vi "Test Flatten to Path.vi"() -> ()   [LabVIEW 2017]
uses:
  c9b6f366-5878-41eb-ba35-ba660d6be02e.vi
  Variant to JSON Text.vi
  JSONtext.lvlib
  <vilib>/addons/_JKI Toolkits/Caraya/classes/Test/Test.lvclass
  <vilib>/addons/_JKI Toolkits/Caraya/classes/Assert/Assert.lvclass
panel:
  out "$Paths":string[](array[string])
  out "<JSON>":string
  out "JSON recovered":bool
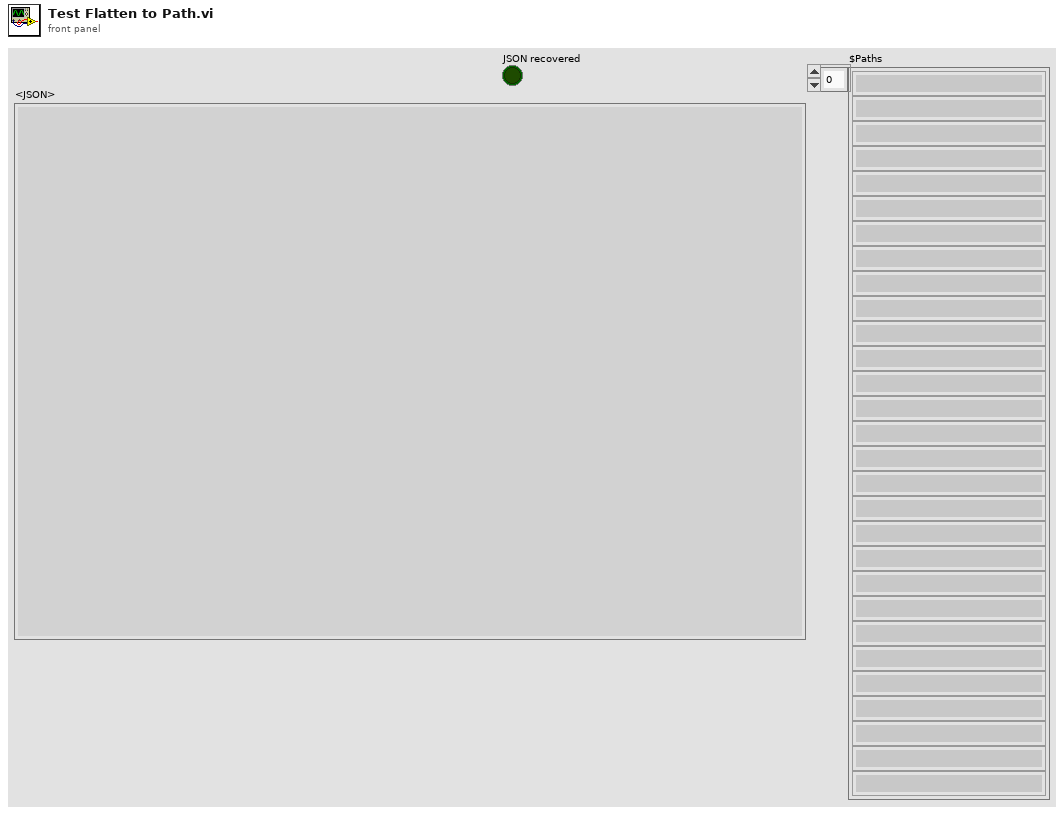
[diagram p1: front panel]
types:
  T1 = cluster{"Number":i32, "String":string, "Timestamp":timestamp, "Reply refnum":refnum<queue>, "VISA resource name":refnum<visa-resource-name>, "True":bool, "Enum":enum16{"Enum 1", "Enum 22", "Enum 333"}, "DBL":dbl, "SubC":cluster{"Number":i32, "String":string, "Timestamp":timestamp, "Reply refnum":refnum<queue>, "VISA resource name":refnum<visa-resource-name>, "True":bool, "Enum":enum16{"Enum 1", "Enum 22", "Enum 333"}, "DBL":dbl, "SubC":cluster{"Number":i32, "String":string, "Timestamp":timestamp, "Reply refnum":refnum<queue>, "VISA resource name":refnum<visa-resource-name>, "True":bool, "Enum":enum16{"Enum 1", "Enum 22", "Enum 333"}, "DBL":dbl}}}
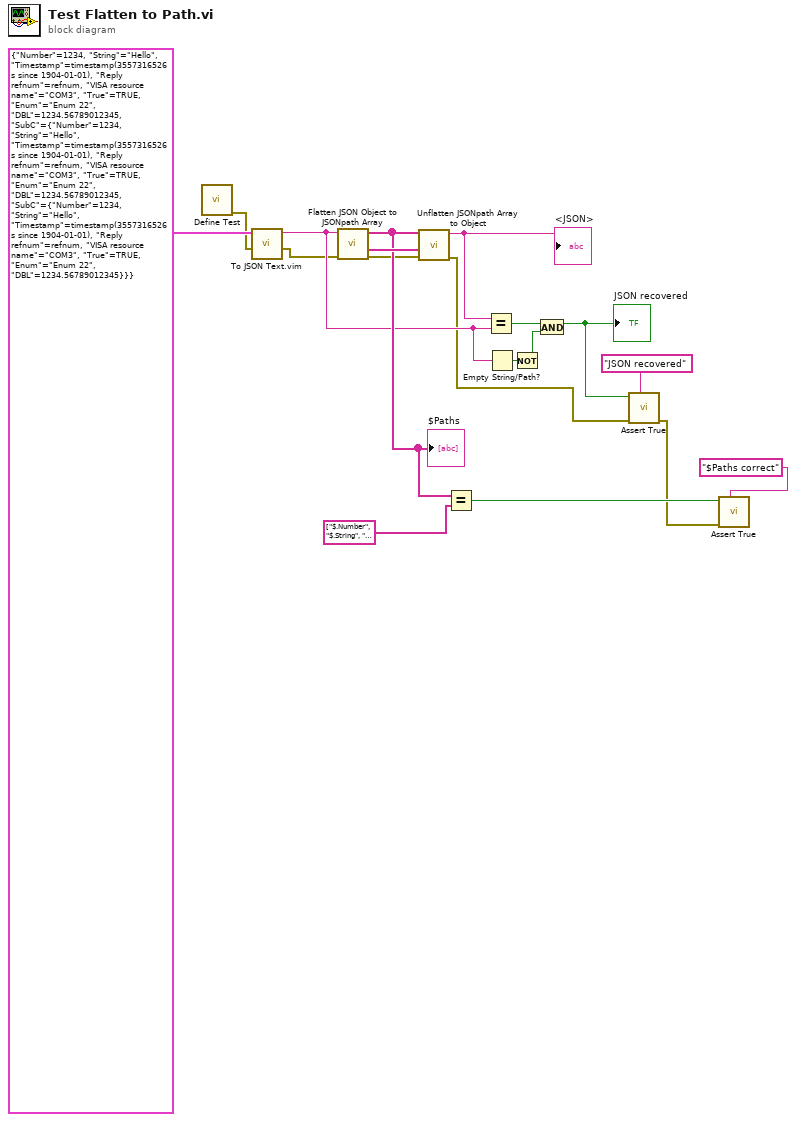
[diagram p0: block diagram]
diagram:
  n1 = call <vilib>:"Define Test.vi"() -> ("error out"=w2:errorcluster)  [unwired: 11 in]
  n2 = call "To JSON Text.vim"("error in (no error)"=w2, "Anything"=T1 {"Number"=1234, "String"="Hello", "Timestamp"=timestamp(3557316526.864 s since 1904-01-01), "Reply refnum"=refnum, "VISA resource name"="COM3", "True"=TRUE, "Enum"=enum."Enum 22", "DBL"=1234.56789012345, "SubC"={"Number"=1234, "String"="Hello", "Timestamp"=timestamp(3557316526.864 s since 1904-01-01), "Reply refnum"=refnum, "VISA resource name"="COM3", "True"=TRUE, "Enum"=enum."Enum 22", "DBL"=1234.56789012345, "SubC"={"Number"=1234, "String"="Hello", "Timestamp"=timestamp(3557316526.864 s since 1904-01-01), "Reply refnum"=refnum, "VISA resource name"="COM3", "True"=TRUE, "Enum"=enum."Enum 22", "DBL"=1234.56789012345}}}) -> ("error out"=w5:errorcluster, "<JSON>"=w12:string)  [unwired: 8 in]
  n3 = call "Flatten JSON Object to JSONpath Array.vi"("error in (no error)"=w5, "JSON"=w12) -> ("error out"=w4:errorcluster, "<JSON>"=w15:string[], "$Paths"=w14:string[])  [unwired: 7 in]
  "$Paths" <- w14
  n4 = call "Unflatten JSONpath Array to Object.vi"("error in (no error)"=w4, "JSON Items"=w15, "$Paths"=w14) -> ("error out"=w3:errorcluster, "<JSON>"=w17:string)  [unwired: 7 in]
  "<JSON>" <- w17
  n5 = Equal?(x=w14, y=string[] ["$.Number", "$.String", "$.Timestamp", "$.Reply refnum", "$.VISA resource name", "$.True", "$.Enum", "$.DBL", "$.SubC.Number", "$.SubC.String", "$.SubC.Timestamp", "$.SubC.Reply refnum", "$.SubC.VISA resource name", "$.SubC.True", "$.SubC.Enum", "$.SubC.DBL", "$.SubC.SubC.Number", "$.SubC.SubC.String", "$.SubC.SubC.Timestamp", "$.SubC.SubC.Reply refnum", "$.SubC.SubC.VISA resource name", "$.SubC.SubC.True", "$.SubC.SubC.Enum", "$.SubC.SubC.DBL"] ("$Paths")) -> (x = y?=w7:bool)
  n6 = Equal?(x=w17, y=w12) -> (x = y?=w16:bool)
  n7 = Empty String/Path?(string/path=w12) -> (empty?=w10:bool)
  n8 = Not(x=w10) -> (.not. x?=w11:bool)
  n9 = And(x=w16, y=w11) -> (x .and. y?=w8:bool)
  "JSON recovered" <- w8
  n10 = call <vilib>:"Assert True.vi"("Label"="JSON recovered", "error in (no error)"=w3, "True?"=w8) -> ("error out"=w1:errorcluster)  [unwired: 8 in]
  n11 = call <vilib>:"Assert True.vi"("Label"="$Paths correct", "error in (no error)"=w1, "True?"=w7) -> ()  [unwired: 8 in, 1 out]
